vi "OpenRectifierLog.vi"(8 "error in (no error)":errorcluster) -> (0 "error out":errorcluster, 3 "Fileref out":refnum<file>)   [LabVIEW 2019]
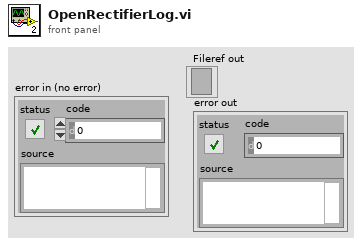
[diagram p1: front panel]
types:
  T1 = enum16{"open", "replace", "create", "open or create", "replace or create", "replace or create with confirmation"}
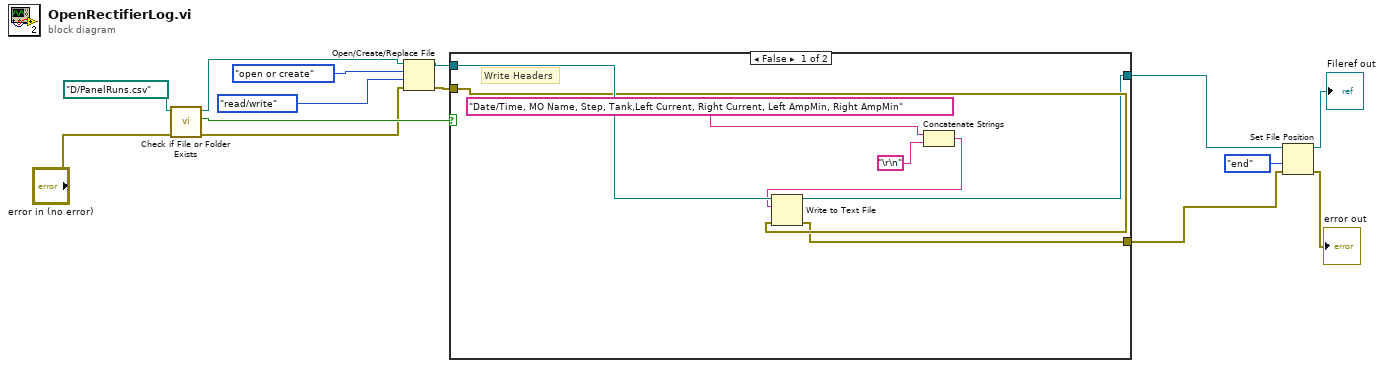
[diagram p0: block diagram]
diagram:
  n1 = call <vilib>:"Check if File or Folder Exists.vi"("error in (no error)"="error in (no error)", "path"=path "D:/PanelRuns.csv" ("file path (use dialog)")) -> ("error out"=w11:errorcluster, "file or folder exists?"=w12:bool, "dup path"=w10:path)  [unwired: 7 in]
  n2 = Open/Create/Replace File(file path (use dialog)=w10, error in=w11, operation (0:open)=T1."open or create", access (0:read/write)=enum16{"read/write", "read-only", "write-only"}."read/write") -> (refnum out=w13:refnum<file>, error out=w14:errorcluster)  [unwired: 2 in, 1 out]
  n3 = case shown="False" w12 {
    tunnel: w13 -> [w21 w23]
    tunnel: w14 -> [w20 w22]
    tunnel: [w19 w22] -> w2
    tunnel: [w18 w23] -> w4
    frame False {
      # "Write Headers"
      n4 = Concatenate Strings("Date/Time, MO Name, Step, Tank,Left Current, Right Current, Left AmpMin, Right AmpMin", "\r\n") -> (w15:string)
      n5 = Write to Text File(file (use dialog)=w21, text=w15, error in=w20) -> (refnum out=w18:refnum<file>, error out=w19:errorcluster)  [unwired: 1 in, 1 out]
    }
    frame True {
    }
  }
  n6 = Set File Position(refnum=w4, from (0:start)=enum16{"start", "end", "current"}."end", error in=w2) -> (refnum out=→"Fileref out":refnum<file>, error out=→"error out":errorcluster)  [unwired: 1 in]
